vi "MindwaveReadByte.vi"(3 "error in (no error) input":errorcluster, 6 "VISA resource name input":refnum<visa-resource-name>) -> (0 "error out":errorcluster, 1 "byte":u8 format="%x", 2 "VISA resource name out":refnum<visa-resource-name>)   [LabVIEW 2011, in "Neurosky.lvlib"]
uses:
  Users/Isaias/Documents/GitHub/Neurosky/Neurosky.lvlib
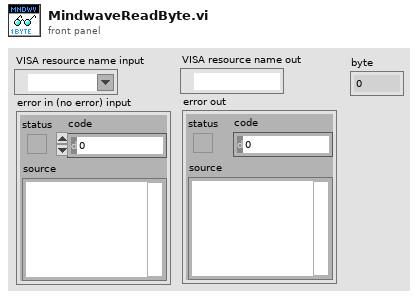
[diagram p1: front panel]
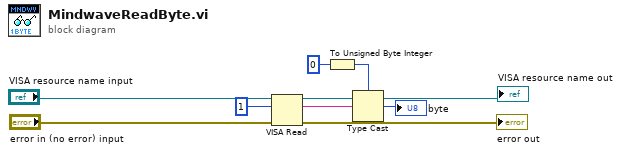
[diagram p0: block diagram]
diagram:
  n1 = VISA Read(VISA resource name="VISA resource name input", byte count=u32 1, error in (no error)="error in (no error) input") -> (VISA resource name out=→"VISA resource name out":refnum<visa-resource-name>, read buffer=w8:string, error out=→"error out":errorcluster)  [unwired: 1 out]
  n2 = To Unsigned Byte Integer(number=i8 0) -> (unsigned 8bit integer=w6:u8)
  n3 = Type Cast(type=w6, x=w8) -> (*(type *) &x=→"byte":u8)
